vi "Pump_API_Test.vi"() -> ()   [LabVIEW 2021]
uses:
  labbCAN_Bus_API/SiUnitPrefix.ctl
  labbCAN_Pump_API/VolumeUnits.ctl
  labbCAN_Bus_API/TimeUnits.ctl
  labbCAN_Bus_API/labbCAN_Bus_API.lvlib
  labbCAN_Pump_API/labbCAN_Pump_API.lvlib
  labbCAN_Valve_API/labbCAN_Valve_API.lvlib
panel:
  out "Syringe Fill Level":dbl
  out "VolumeMax":dbl
  out "FlowRateMax":dbl
  out "Valve position":i32
  out "Valve positions":i32
  out "Has valve":bool
  out "Calibration finished":bool
  out "error out":errorcluster caption="Fehler (Ausgang)"
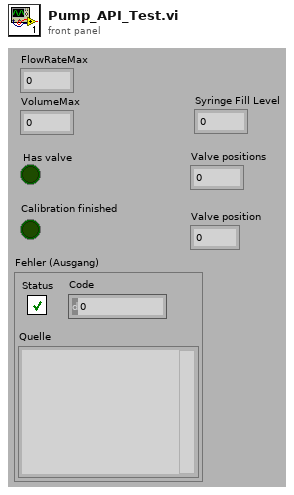
[diagram p1: front panel]
types:
  T1 = typedef "labbCAN_Bus_API.lvlib/TimeUnits.ctl" = i32
  T2 = typedef "labbCAN_Pump_API.lvlib/VolumeUnits.ctl" = i32
  T3 = typedef "labbCAN_Bus_API.lvlib/SiUnitPrefix.ctl" = i32
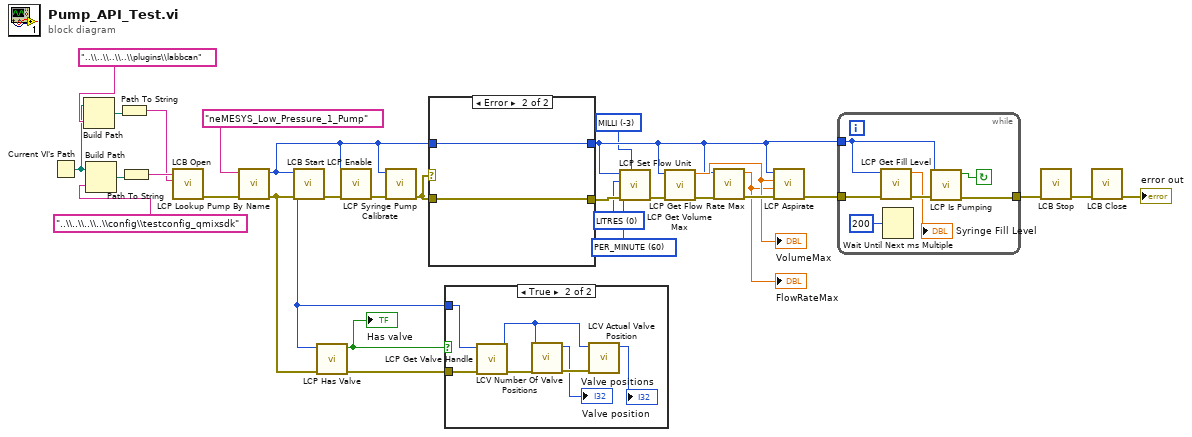
[diagram p0: block diagram]
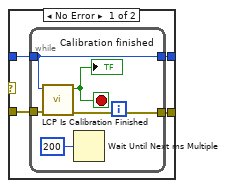
[diagram p2: hidden frame]
diagram:
  w6 = T1 60 items=["PER_SECOND"=1, "PER_MINUTE"=60, "PER_HOUR"=3600] ("TimeUnit")
  w7 = T2 0 items=["LITRES"] ("VolumeUnit")
  w8 = T3 -3 items=["UNIT"=0, "DECI"=-1, "CENTI"=-2, "MILLI"=-3, "MICRO"=-6] ("Prefix")
  n1 = Current VI's Path() -> (path=w3:path)
  n2 = Build Path(base path=w3, name or relative path="..\\..\\..\\..\\plugins\\labbcan" ("Name oder relativer Pfad")) -> (appended path=w5:path)
  n3 = Build Path(base path=w3, name or relative path="..\\..\\..\\..\\config\\testconfig_qmixsdk" ("Name oder relativer Pfad")) -> (appended path=w18:path)
  n4 = Path To String(path=w5) -> (string=w2:string)
  n5 = Path To String(path=w18) -> (string=w16:string)
  n6 = call "LCB Open.vi"("PluginSearchPath"=w2, "Device Configuration Path"=w16) -> ("error out"=w29:errorcluster)  [unwired: 9 in]
  n7 = call "LCP Lookup Pump By Name.vi"("error in (no error)"=w29, "Pump Name"="neMESYS_Low_Pressure_1_Pump" ("pAxisName")) -> ("error out"=w23:errorcluster, "Pump handle"=w21:i64)  [unwired: 8 in]
  n8 = call "LCB Start.vi"("error in (no error)"=w23) -> ("error out"=w26:errorcluster)  [unwired: 10 in]
  n9 = call "LCP Has Valve.vi"("error in (no error)"=w23, "Pump Handle"=w21) -> ("error out"=w22:errorcluster, "Has Valve"=w24:bool)  [unwired: 8 in]
  "Has valve" <- w24
  n10 = call "LCP Enable.vi"("error in (no error)"=w26, "Pump Handle"=w21) -> ("error out"=w25:errorcluster)  [unwired: 9 in]
  n11 = call "LCP Syringe Pump Calibrate.vi"("error in (no error)"=w25, "Pump Handle"=w21) -> ("error out"=w1:errorcluster)  [unwired: 9 in]
  n12 = case shown="Error" w1 {
    tunnel: w1 -> [w34 w41]
    tunnel: w21 -> [w33 w40]
    tunnel: [w32 w41] -> w10
    tunnel: [w31 w40] -> w9
    frame No Error {
      n13 = while {
        tunnel: w34 -> [w37]
        tunnel: w33 -> [w36]
        tunnel: [w39] -> w32
        tunnel: [w36] -> w31
        stop <- w35 stop-if-true
        n14 = call "LCP Is Calibration Finished.vi"("error in (no error)"=w37, "Pump Handle"=w36) -> ("error out"=w39:errorcluster, "Calibration Finished"=w35:bool)  [unwired: 8 in]
        "Calibration finished" <- w35
        n15 = Wait Until Next ms Multiple(millisecond multiple=u32 200 ("Vielfache von ms")) -> ()  [unwired: 1 out]
      }
    }
    frame Error {
    }
  }
  n16 = case shown="True" w24 {
    tunnel: w22 -> [_ w48]
    tunnel: w21 -> [_ w45]
    frame False {
    }
    frame True {
      n17 = call "LCP Get Valve Handle.vi"("error in (no error)"=w48, "Pump Handle"=w45) -> ("error out"=w47:errorcluster, "Valve Handle"=w44:i64)  [unwired: 8 in]
      n18 = call "LCV Number Of Valve Positions.vi"("error in (no error)"=w47, "Valve Handle"=w44) -> ("error out"=w46:errorcluster, "Valve Position Count"=→"Valve positions":i32)  [unwired: 8 in]
      n19 = call "LCV Actual Valve Position.vi"("error in (no error)"=w46, "Valve Handle"=w44) -> ("Actual valve position"=→"Valve position":i32)  [unwired: 8 in, 1 out]
    }
  }
  n20 = call "LCP Set Flow Unit.vi"("Prefix"=w8, "error in (no error)"=w10, "TimeUnit"=w6, "VolumeUnit"=w7, "Pump Handle"=w9) -> ("error out"=w11:errorcluster)  [unwired: 6 in]
  n21 = call "LCP Get Volume Max.vi"("error in (no error)"=w11, "Pump Handle"=w9) -> ("error out"=w15:errorcluster, "Maximum Volume"=w13:dbl)  [unwired: 8 in]
  "VolumeMax" <- w13
  n22 = call "LCP Get Flow Rate Max.vi"("error in (no error)"=w15, "Pump Handle"=w9) -> ("error out"=w14:errorcluster, "Maximum Flow Rate"=w12:dbl)  [unwired: 8 in]
  "FlowRateMax" <- w12
  n23 = call "LCP Aspirate.vi"("error in (no error)"=w14, "Flow"=w12, "Volume"=w13, "Pump Handle"=w9) -> ("error out"=w20:errorcluster)  [unwired: 7 in]
  n24 = while {
    tunnel: w20 -> [w52]
    tunnel: w9 -> [w50]
    tunnel: [w53] -> w19
    stop <- w54 continue-if-true
    n25 = call "LCP Get Fill Level.vi"("error in (no error)"=w52, "Pump Handle"=w50) -> ("error out"=w51:errorcluster, "Fill Level"=→"Syringe Fill Level":dbl)  [unwired: 8 in]
    n26 = Wait Until Next ms Multiple(millisecond multiple=u32 200 ("Vielfache von ms")) -> ()  [unwired: 1 out]
    n27 = call "LCP Is Pumping.vi"("error in (no error)"=w51, "Pump Handle"=w50) -> ("error out"=w53:errorcluster, "Is pumping"=w54:bool)  [unwired: 8 in]
  }
  n28 = call "LCB Stop.vi"("error in (no error)"=w19) -> ("error out"=w27:errorcluster)  [unwired: 10 in]
  n29 = call "LCB Close.vi"("error in (no error)"=w27) -> ("error out"=→"error out":errorcluster)  [unwired: 10 in]
